vi "Test_WindowFrame.vi"() -> ()   [LabVIEW 2021]
uses:
  WindowFrame.lvclass
  FrontPanel.Run-TimePosition.GetPosition.ctl
  <vilib>/Utility/miscctls.llb/LVPointTypeDef.ctl
  <vilib>/Utility/miscctls.llb/LVRectTypeDef.ctl
panel:
  in  "Update Properties":bool
  in  "All Properties":T3={"Allow Runtime PopUp"=FALSE, "Behavior"=enum."Invalid", "Closable"=FALSE, "Custom Title"=FALSE, "Highlight Return Button"=FALSE, "Is Frontmost"=FALSE, "Minimizable"=FALSE, "Minimum Size"={"Horizontal"=0, "Vertical"=0}, "Monitor"=0, "Panel Bounds"={"Left"=0, "Top"=0, "Right"=500, "Bottom"=500}, "Resizable"=FALSE, "Run VI Transparently"=FALSE, "Show Menu Bar"=FALSE, "State"=enum."Standard", "Title"="TEST WINDOW FRAME 1", "Title Bar Colors [4]"=[{9868950, 9868950}, {13816530, 13816530}, {9868950, 9868950}, {13816530, 13816530}], "Title Bar Visible"=FALSE, "Transparancy"=0, "Window Bounds"={"Left"=0, "Top"=0, "Right"=500, "Bottom"=500}}
  in  "Read Properties":bool
  out "GetPosition":T4
  in  "Run-Time Position.Get Position 1":bool
  in  "Size 3":cluster{"Height":i16, "Width":i16}
  in  "Position":cluster{"Top":i16, "Left":i16}
  in  "Run-Time Position.Custom 1":bool
  in  "Center Window Frame 1":bool
  in  "Size":cluster{"Height":i16, "Width":i16}
  in  "Monitor":i16
  in  "Run-Time Position.Centered 1":bool
  in  "Close Window Frame 1":bool
  in  "State 2":T5(ring)=enum."Standard"
  in  "State 1":T5(ring)=enum."Standard"
  in  "Open Window Frame 2":bool
  in  "Open Window Frame 1":bool
  out "WindowFrameClose 1":bool
  out "WindowFrameClose 2":bool
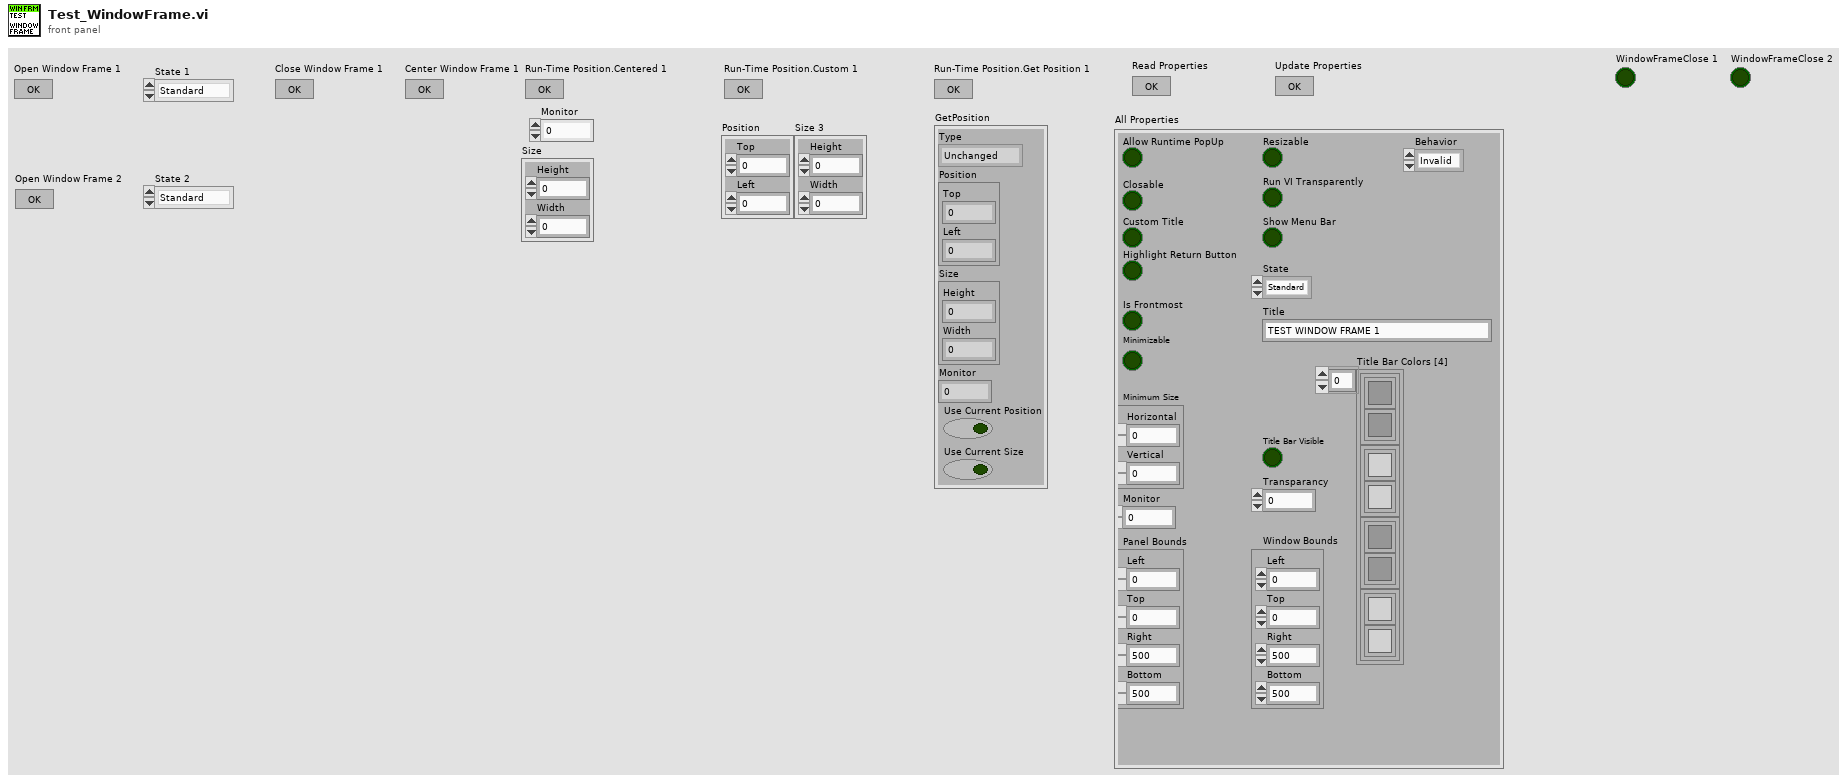
[diagram p1: front panel]
types:
  T1 = typedef "LVPointTypeDef.ctl" = cluster{"Horizontal":i16, "Vertical":i16}
  T2 = typedef "LVRectTypeDef.ctl" = cluster{"Left":i16, "Top":i16, "Right":i16, "Bottom":i16}
  T3 = cluster{"Allow Runtime PopUp":bool, "Behavior":enum32{"Invalid", "Default", "Floating", "Floating/Auto-Hide", "Modal"}, "Closable":bool, "Custom Title":bool, "Highlight Return Button":bool, "Is Frontmost":bool, "Minimizable":bool, "Minimum Size":T1, "Monitor":u16, "Panel Bounds":T2, "Resizable":bool, "Run VI Transparently":bool, "Show Menu Bar":bool, "State":enum32{"Invalid", "Standard", "Closed", "Hidden", "Minimized", "Maximized"}, "Title":string, "Title Bar Colors [4]":cluster{u32, u32}[], "Title Bar Visible":bool, "Transparancy":u8, "Window Bounds":T2}
  T4 = typedef "WindowFrame.lvlib/WindowFrame.lvclass/FrontPanel.Run-TimePosition.GetPosition.ctl" = cluster{"Type":enum32{"Unchanged", "Centered", "Maximized", "Minimized", "Custom"}, "Position":cluster{"Top":i16, "Left":i16}, "Size":cluster{"Height":i16, "Width":i16}, "Monitor":i16, "Use Current Position":bool, "Use Current Size":bool}
  T5 = enum32{"Invalid", "Standard", "Closed", "Hidden", "Minimized", "Maximized"}
  T6 = cluster{"WF1":refnum<event-registration>, "WF2":refnum<event-registration>}
  T7 = enum32{"Invalid", "Default", "Floating", "Floating/Auto-Hide", "Modal"}
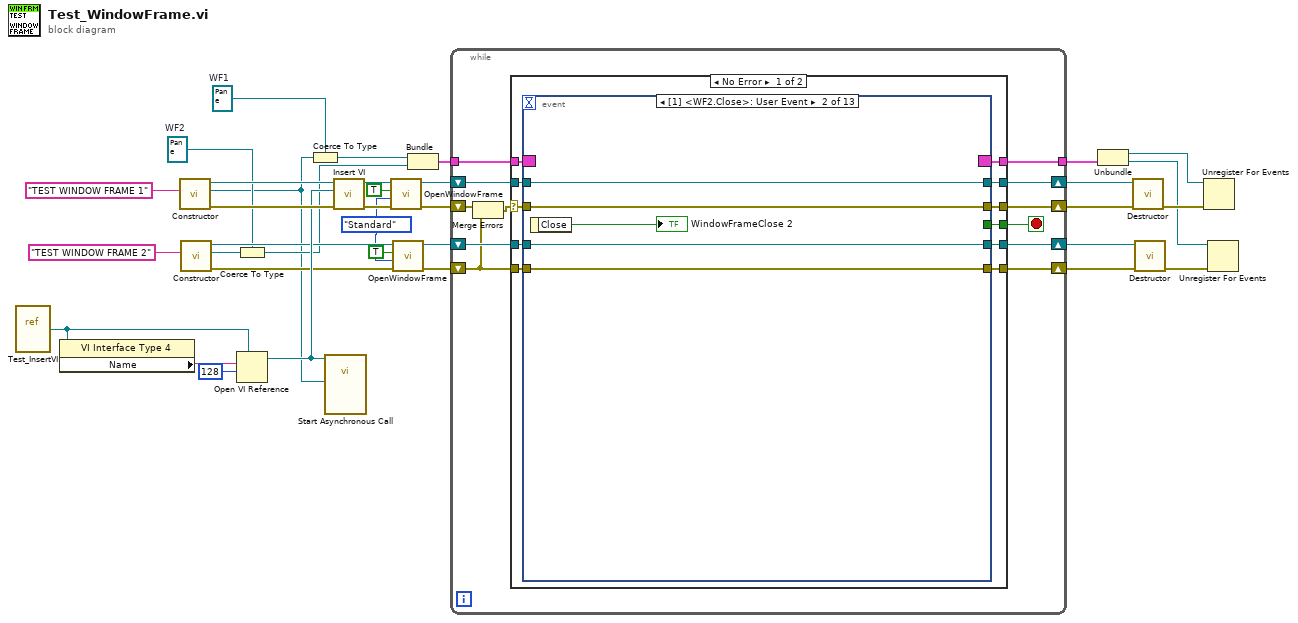
[diagram p0: block diagram]
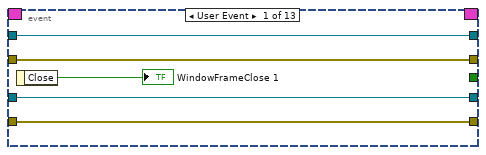
[diagram p2: hidden frame]
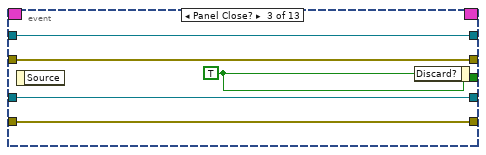
[diagram p3: hidden frame]
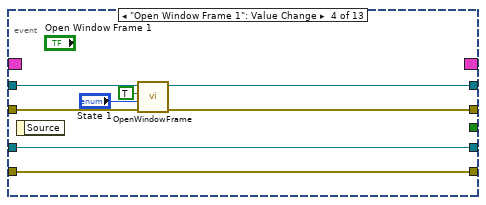
[diagram p4: hidden frame]
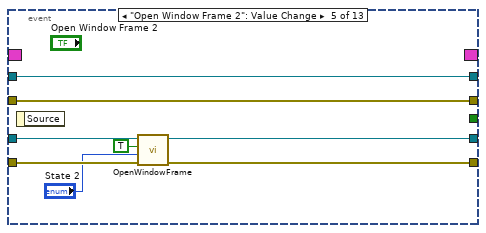
[diagram p5: hidden frame]
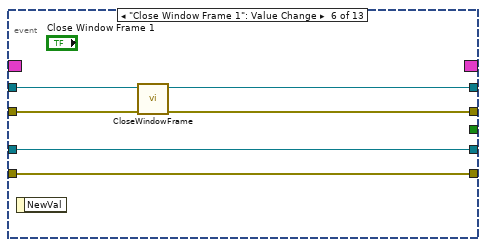
[diagram p6: hidden frame]
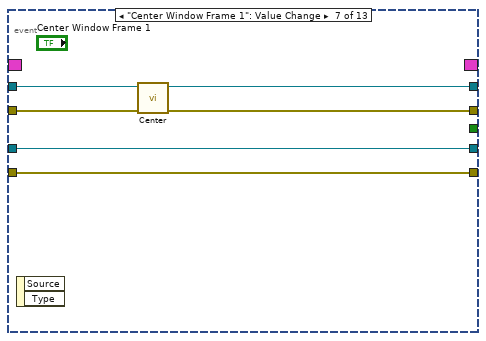
[diagram p7: hidden frame]
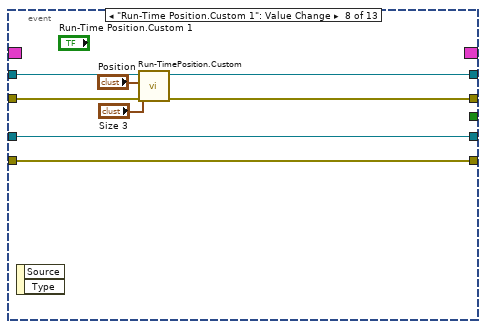
[diagram p8: hidden frame]
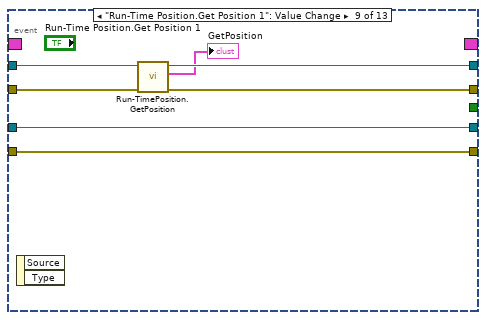
[diagram p9: hidden frame]
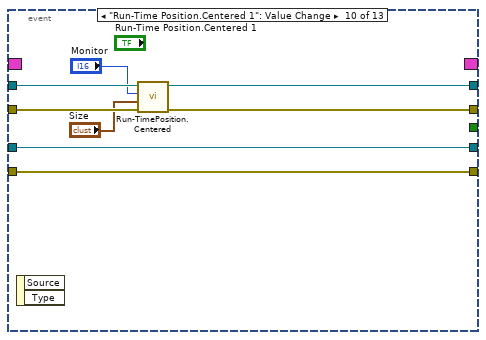
[diagram p10: hidden frame]
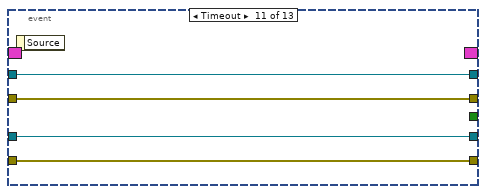
[diagram p11: hidden frame]
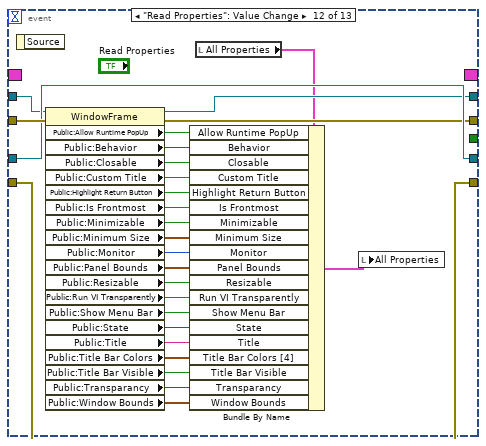
[diagram p12: hidden frame]
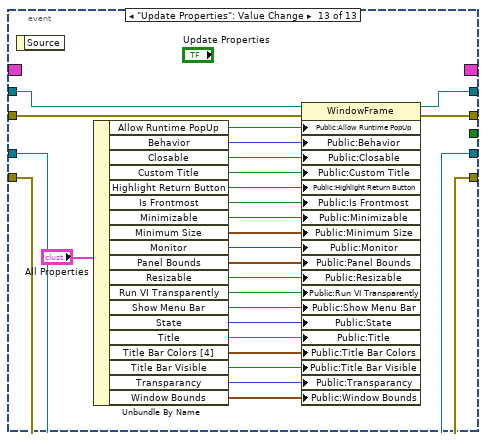
[diagram p13: hidden frame]
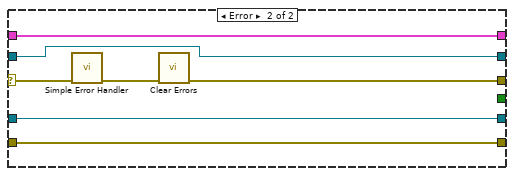
[diagram p14: hidden frame]
diagram:
  w3 = refnum<event-registration> refnum  # WF2
  w5 = refnum<event-registration> refnum  # WF1
  w8 = T5."Standard" ("State")
  n1 = vi-ref "Test_InsertVI.vi"() -> (w21:refnum<vi>)
  n2 = property class="VI Interface Type 4"(reference=w21) -> ("Name"=w20:string)  [unwired: 1 in, 2 out]
  n3 = call "Constructor.vi"("WindowTitle"="TEST WINDOW FRAME 1") -> ("error out"=w34:errorcluster, "WindowFrame"=w1:refnum<event-registration>, "WindowFrame out"=w17:refnum<class "WindowFrame.lvclass">)  [unwired: 8 in]
  n4 = call "Constructor.vi"("WindowTitle"="TEST WINDOW FRAME 2") -> ("error out"=w10:errorcluster, "WindowFrame"=w30:refnum<event-registration>, "WindowFrame out"=w12:refnum<class "WindowFrame.lvclass">)  [unwired: 8 in]
  n5 = Coerce To Type(0:w30, 1:w3) -> (2:w4:refnum<event-registration>)
  n6 = Open VI Reference(type specifier VI Refnum (for type only)=w21, vi path=w20, options=128) -> (vi reference=w16:refnum<vi>)  [unwired: 3 in, 1 out]
  n7 = Coerce To Type(0:w1, 1:w5) -> (2:w2:refnum<event-registration>)
  n8 = call-by-ref "Start Asynchronous Call"(reference=w16, "WF1"=w1) -> ()  [unwired: 12 in, 2 out]
  n9 = call "Insert VI.vi"("error in (no error)"=w34, "VI Refnum"=w16, "WindowFrame in"=w17) -> ("error out"=w18:errorcluster, "WindowFrame out"=w14:refnum<class "WindowFrame.lvclass">)  [unwired: 7 in]
  n10 = call "OpenWindowFrame.vi"("error in (no error)"=w18, "State"=w8, "Activate?"=TRUE, "WindowFrame in"=w14) -> ("error out"=w15:errorcluster, "WindowFrame out"=w13:refnum<class "WindowFrame.lvclass">)  [unwired: 6 in]
  n11 = call "OpenWindowFrame.vi"("error in (no error)"=w10, "State"=w8, "Activate?"=TRUE, "WindowFrame in"=w12) -> ("error out"=w9:errorcluster, "WindowFrame out"=w11:refnum<class "WindowFrame.lvclass">)  [unwired: 6 in]
  n12 = Bundle("WF1"=w2, "WF2"=w4) -> (w33:T6)  [unwired: 1 in]
  n13 = while {
    tunnel: w33 -> [w47]
    shift-right: [w44] -> w27
    shift-left: w13 -> [w45]
    shift-right: [w37] -> w32
    shift-left: w15 -> [w46]
    shift-right: [w40] -> w29
    shift-left: w11 -> [w41]
    shift-right: [w36] -> w28
    shift-left: w9 -> [w38]
    tunnel: [w39] -> w26
    stop <- w43 stop-if-true
    n14 = Merge Errors(w46, w38) -> (w42:errorcluster)
    n15 = case shown="No Error" w42 {
      selector: w42 -> [w57 w188]
      tunnel: w47 -> [w58 w185]
      tunnel: [w56 w186] -> w37
      tunnel: w45 -> [w55 w184]
      tunnel: [w54 w184] -> w44
      tunnel: [w53 _] -> w43
      tunnel: w41 -> [w52 w183]
      tunnel: [w51 w183] -> w40
      tunnel: [w50 w185] -> w39
      tunnel: w38 -> [w49 w182]
      tunnel: [w48 w182] -> w36
      frame No Error {
        n16 = event shown="[1] <WF2.Close>: User Event" {
          selector: w58 -> [_ _ _ _ _ _ _ _ _ _ _ _ _]
          dyn-events: [_ _ _ _ _ _ _ _ _ _ _ _ _] -> w50
          timeout: _ -> [_ _ _ _ _ _ _ _ _ _ _ _ _]
          tunnel: [w63 w66 w73 w78 w89 w92 w98 w106 w113 w121 w127 w152 w178] -> w56
          tunnel: w57 -> [w63 w66 w73 w81 w89 w95 w101 w109 w116 w124 w127 w155 w181]
          tunnel: [w62 w67 w70 w76 w88 w90 w96 w104 w111 w119 w128 w150 w176] -> w54
          tunnel: w55 -> [w62 w67 w70 w77 w88 w91 w97 w105 w112 w120 w128 w151 w177]
          tunnel: [_ _ w71 _ _ _ _ _ _ _ _ _ _] -> w53
          tunnel: w52 -> [w61 w65 w72 w80 w85 w94 w100 w108 w115 w123 w126 w154 w180]
          tunnel: [w61 w65 w72 w80 w84 w94 w100 w108 w115 w123 w126 w154 w180] -> w51
          tunnel: w49 -> [w59 w64 w69 w79 w87 w93 w99 w107 w114 w122 w125 w153 w179]
          tunnel: [w59 w64 w69 w79 w86 w93 w99 w107 w114 w122 w125 w153 w179] -> w48
          event User Event {
            n17 = event-data() -> ("Close"=→"WindowFrameClose 1":bool)  [unwired: 1 in]
          }
          event User Event {
            n18 = event-data() -> ("Close"=→"WindowFrameClose 2":bool)  [unwired: 1 in]
          }
          event Panel Close? {
            w71 = TRUE ("Discard?")
            n19 = event-data() -> ()  [unwired: 1 in, 1 out]
            n20 = event-data("Discard?"=w71) -> ()  [unwired: 1 in, 1 out]
          }
          event "Open Window Frame 1": Value Change {
            n21 = event-data() -> ()  [unwired: 1 in, 1 out]
            n22 = call "OpenWindowFrame.vi"("error in (no error)"=w81, "State"="State 1", "Activate?"=TRUE, "WindowFrame in"=w77) -> ("error out"=w78:errorcluster, "WindowFrame out"=w76:refnum<class "WindowFrame.lvclass">)  [unwired: 6 in]
          }
          event "Open Window Frame 2": Value Change {
            n23 = event-data() -> ()  [unwired: 1 in, 1 out]
            n24 = call "OpenWindowFrame.vi"("error in (no error)"=w87, "State"="State 2", "Activate?"=TRUE, "WindowFrame in"=w85) -> ("error out"=w86:errorcluster, "WindowFrame out"=w84:refnum<class "WindowFrame.lvclass">)  [unwired: 6 in]
          }
          event "Close Window Frame 1": Value Change {
            n25 = event-data() -> ()  [unwired: 1 in, 1 out]
            n26 = call "CloseWindowFrame.vi"("error in (no error)"=w95, "WindowFrame in"=w91) -> ("error out"=w92:errorcluster, "WindowFrame out"=w90:refnum<class "WindowFrame.lvclass">)  [unwired: 8 in]
          }
          event "Center Window Frame 1": Value Change {
            n27 = event-data() -> ()  [unwired: 1 in, 2 out]
            n28 = call "Center.vi"("error in (no error)"=w101, "WindowFrame in"=w97) -> ("error out"=w98:errorcluster, "WindowFrame out"=w96:refnum<class "WindowFrame.lvclass">)  [unwired: 8 in]
          }
          event "Run-Time Position.Custom 1": Value Change {
            n29 = event-data() -> ()  [unwired: 1 in, 2 out]
            n30 = call "Run-TimePosition.Custom.vi"("error in (no error)"=w109, "Size"="Size 3", "Position"="Position", "WindowFrame in"=w105) -> ("error out"=w106:errorcluster, "WindowFrame out"=w104:refnum<class "WindowFrame.lvclass">)  [unwired: 6 in]
          }
          event "Run-Time Position.Get Position 1": Value Change {
            n31 = event-data() -> ()  [unwired: 1 in, 2 out]
            n32 = call "Run-TimePosition.GetPosition.vi"("error in (no error)"=w116, "WindowFrame in"=w112) -> ("error out"=w113:errorcluster, "GetPosition"=→"GetPosition":T4, "WindowFrame out"=w111:refnum<class "WindowFrame.lvclass">)  [unwired: 7 in]
          }
          event "Run-Time Position.Centered 1": Value Change {
            n33 = event-data() -> ()  [unwired: 1 in, 2 out]
            n34 = call "Run-TimePosition.Centered.vi"("error in (no error)"=w124, "Size"="Size", "Monitor"="Monitor", "WindowFrame in"=w120) -> ("error out"=w121:errorcluster, "WindowFrame out"=w119:refnum<class "WindowFrame.lvclass">)  [unwired: 6 in]
          }
          event Timeout {
            n35 = event-data() -> ()  [unwired: 1 in, 1 out]
          }
          event "Read Properties": Value Change {
            n36 = event-data() -> ()  [unwired: 1 in, 1 out]
            n37 = property class="WindowFrame"(reference=w151, error in=w155) -> (reference out=w150:refnum<class "WindowFrame.lvclass">, error out=w152:errorcluster, "Public:Allow Runtime PopUp"=w130:bool, "Public:Behavior"=w129:T7, "Public:Closable"=w131:bool, "Public:Custom Title"=w132:bool, "Public:Highlight Return Button"=w133:bool, "Public:Is Frontmost"=w134:bool, "Public:Minimizable"=w135:bool, "Public:Minimum Size"=w136:T1, "Public:Monitor"=w137:u16, "Public:Panel Bounds"=w138:T2, "Public:Resizable"=w139:bool, "Public:Run VI Transparently"=w140:bool, "Public:Show Menu Bar"=w141:bool, "Public:State"=w142:T5, "Public:Title"=w143:string, "Public:Title Bar Colors"=w144:cluster{u32, u32}[], "Public:Title Bar Visible"=w145:bool, "Public:Transparancy"=w146:u8, "Public:Window Bounds"=w147:T2)
            n38 = local read "All Properties"() -> (w149:T3)
            n39 = Bundle By Name(cluster=w149, "Allow Runtime PopUp"=w130, "Behavior"=w129, "Closable"=w131, "Custom Title"=w132, "Highlight Return Button"=w133, "Is Frontmost"=w134, "Minimizable"=w135, "Minimum Size"=w136, "Monitor"=w137, "Panel Bounds"=w138, "Resizable"=w139, "Run VI Transparently"=w140, "Show Menu Bar"=w141, "State"=w142, "Title"=w143, "Title Bar Colors [4]"=w144, "Title Bar Visible"=w145, "Transparancy"=w146, "Window Bounds"=w147) -> (w148:T3)
            n40 = local write "All Properties"(w148) -> ()
          }
          event "Update Properties": Value Change {
            n41 = event-data() -> ()  [unwired: 1 in, 1 out]
            n42 = Unbundle By Name("All Properties") -> ("Allow Runtime PopUp"=w175:bool, "Behavior"=w156:T7, "Closable"=w174:bool, "Custom Title"=w173:bool, "Highlight Return Button"=w172:bool, "Is Frontmost"=w171:bool, "Minimizable"=w170:bool, "Minimum Size"=w169:T1, "Monitor"=w168:u16, "Panel Bounds"=w167:T2, "Resizable"=w166:bool, "Run VI Transparently"=w165:bool, "Show Menu Bar"=w164:bool, "State"=w163:T5, "Title"=w162:string, "Title Bar Colors [4]"=w161:cluster{u32, u32}[], "Title Bar Visible"=w160:bool, "Transparancy"=w159:u8, "Window Bounds"=w158:T2)
            n43 = property class="WindowFrame"(reference=w177, error in=w181, "Public:Allow Runtime PopUp"=w175, "Public:Behavior"=w156, "Public:Closable"=w174, "Public:Custom Title"=w173, "Public:Highlight Return Button"=w172, "Public:Is Frontmost"=w171, "Public:Minimizable"=w170, "Public:Minimum Size"=w169, "Public:Monitor"=w168, "Public:Panel Bounds"=w167, "Public:Resizable"=w166, "Public:Run VI Transparently"=w165, "Public:Show Menu Bar"=w164, "Public:State"=w163, "Public:Title"=w162, "Public:Title Bar Colors"=w161, "Public:Title Bar Visible"=w160, "Public:Transparancy"=w159, "Public:Window Bounds"=w158) -> (reference out=w176:refnum<class "WindowFrame.lvclass">, error out=w178:errorcluster)
          }
        }
      }
      frame Error {
        n44 = call <vilib>:"Simple Error Handler.vi"("error in (no error)"=w188) -> ("error out"=w187:errorcluster)  [unwired: 4 in, 4 out]
        n45 = call <vilib>:"Clear Errors.vi"("error in (no error)"=w187) -> ("error out"=w186:errorcluster)  [unwired: 5 in, 1 out]
      }
    }
  }
  n46 = Unbundle(w26) -> ("WF1"=w24:refnum<event-registration>, "WF2"=w23:refnum<event-registration>)
  n47 = call "Destructor.vi"("error in (no error)"=w32, "WindowFrame in"=w27) -> ("error out"=w25:errorcluster)  [unwired: 9 in]
  n48 = call "Destructor.vi"("error in (no error)"=w28, "WindowFrame in"=w29) -> ("error out"=w22:errorcluster)  [unwired: 9 in]
  n49 = Unregister For Events(event registration refnum=w24, error in=w25) -> ()  [unwired: 1 out]
  n50 = Unregister For Events(event registration refnum=w23, error in=w22) -> ()  [unwired: 1 out]
